vi "custom_operation_461nm_freq.vi"(10 "Channel":T1={"Operation"=0, "Num. Steps"=0, "Begin"=0.0, "Step Size"=0.0, "Input - A"=0, "Input - B"=0, "Output - LO"=0.0, "Output - HI"=0.0, "Reset"=FALSE, "Analog Output"=0, "Trigger Input"=0, "Initialize To"=0, "Digital Inputs"=[0, 0, 0, 0, 0], "Output Values"=[0.0, 0.0, 0.0, 0.0, 0.0], "Num. Inputs"=4} {"Digital Inputs" items=["DIO0", "DIO1", "DIO2", "DIO3", "DIO4", "DIO5", "DIO6", "DIO7", "DIO8", "DIO9", "DIO10", "DIO11", "DIO12", "DIO13", "DIO14", "DIO15", "DIO16", "DIO17", "DIO18", "DIO19", "DIO20", "DIO21", "DIO22", "DIO23", "DIO24", "DIO25", "DIO26", "DIO27", "DIO28", "DIO29", "DIO30", "DIO31"]; "Initialize To" items=["Zero", "Begin Value"]; "Trigger Input" items=["DIO0", "DIO1", "DIO2", "DIO3", "DIO4", "DIO5", "DIO6", "DIO7", "DIO8", "DIO9", "DIO10", "DIO11", "DIO12", "DIO13", "DIO14", "DIO15", "DIO16", "DIO17", "DIO18", "DIO19", "DIO20", "DIO21", "DIO22", "DIO23", "DIO24", "DIO25", "DIO26", "DIO27", "DIO28", "DIO29", "DIO30", "DIO31"]; "Analog Output" items=["AO\\00", "AO\\01", "AO\\02", "AO\\03", "AO\\04", "AO\\05", "AO\\06", "AO\\07", "AO\\08", "AO\\09", "AO\\10", "AO\\11", "AO\\12", "AO\\13", "AO\\14", "AO\\15"]; "Input - B" items=["DIO0", "DIO1", "DIO2", "DIO3", "DIO4", "DIO5", "DIO6", "DIO7", "DIO8", "DIO9", "DIO10", "DIO11", "DIO12", "DIO13", "DIO14", "DIO15", "DIO16", "DIO17", "DIO18", "DIO19", "DIO20", "DIO21", "DIO22", "DIO23", "DIO24", "DIO25", "DIO26", "DIO27", "DIO28", "DIO29", "DIO30", "DIO31"]; "Input - A" items=["DIO0", "DIO1", "DIO2", "DIO3", "DIO4", "DIO5", "DIO6", "DIO7", "DIO8", "DIO9", "DIO10", "DIO11", "DIO12", "DIO13", "DIO14", "DIO15", "DIO16", "DIO17", "DIO18", "DIO19", "DIO20", "DIO21", "DIO22", "DIO23", "DIO24", "DIO25", "DIO26", "DIO27", "DIO28", "DIO29", "DIO30", "DIO31"]; "Operation" items=["OFF", "SWITCH", "AND GATE", "OR GATE", "ITERATION", "CUSTOM - 461nm Freq."]}, 11 "Digital Input Value Array":bool[](array[boolean])=[FALSE, FALSE, FALSE, FALSE, FALSE, FALSE, FALSE, FALSE, FALSE, FALSE, FALSE, FALSE, FALSE, FALSE, FALSE, FALSE, FALSE, FALSE, FALSE, FALSE, FALSE, FALSE, FALSE, FALSE, FALSE, FALSE, FALSE, FALSE, FALSE, FALSE, FALSE, FALSE]) -> (3 "AO Out":fxp<+/-,20,5>)   [LabVIEW 2016]
uses:
  fpga_array_element.ctl
panel:
  # "Boolean Operation Controls"
  # "Iteration Operation Controls"
  # "Custom Operation Controls"
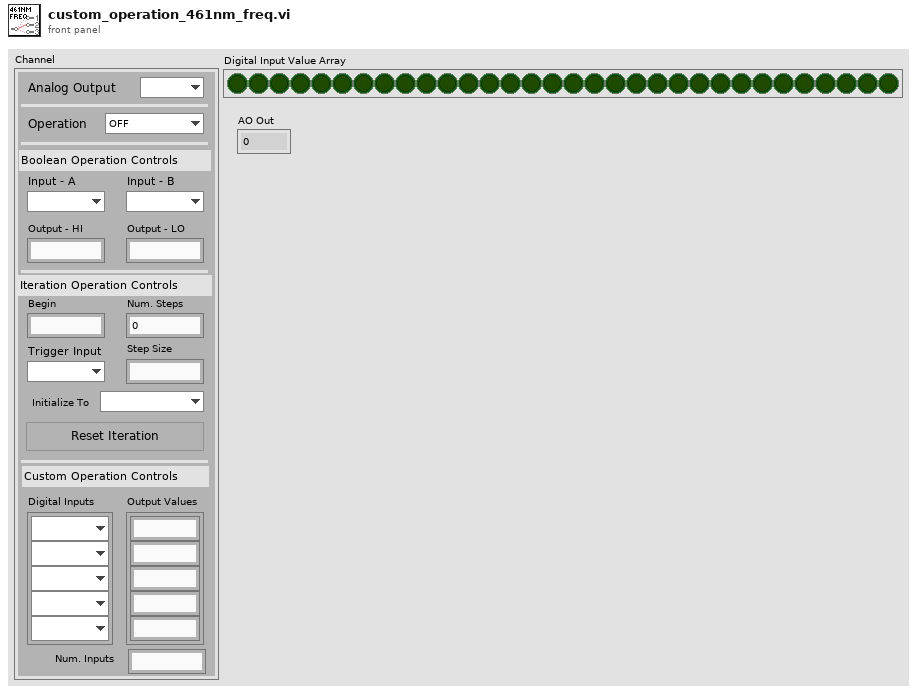
[diagram p1: front panel]
types:
  T1 = typedef "fpga_array_element.ctl" = cluster{"Operation":i16, "Num. Steps":u16, "Begin":fxp<+/-,20,5>, "Step Size":fxp<+/-,20,5>, "Input - A":i32, "Input - B":i32, "Output - LO":fxp<+/-,20,5>, "Output - HI":fxp<+/-,20,5>, "Reset":bool, "Analog Output":i32, "Trigger Input":i32, "Initialize To":i16, "Digital Inputs":i32[], "Output Values":fxp<+/-,20,5>[], "Num. Inputs":u16}
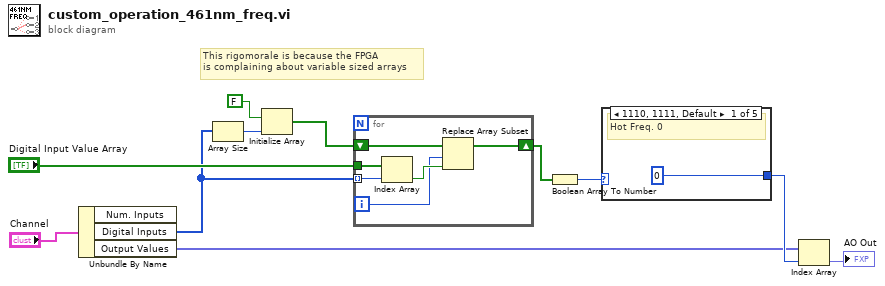
[diagram p0: block diagram]
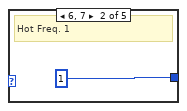
[diagram p2: hidden frame]
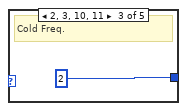
[diagram p3: hidden frame]
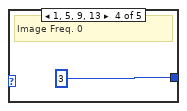
[diagram p4: hidden frame]
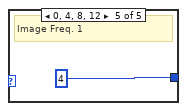
[diagram p5: hidden frame]
diagram:
  # "This rigomorale is because the FPGA\nis complaining about variable sized arrays"
  n1 = Unbundle By Name("Channel") -> ("Digital Inputs"=w5:i32[], "Output Values"=w7:fxp<+/-,20,5>[])  [unwired: 1 out]
  n2 = Array Size(array=w5) -> (size(s)=w4:i32)
  n3 = Initialize Array(FALSE, w4) -> (w2:bool[])
  n4 = for {
    tunnel: "Digital Input Value Array" -> [w17]
    tunnel: w5 -> [w16] mode=indexing
    shift-right: [w12] -> w1
    shift-left: w2 -> [w13]
    i -> [w14]
    n5 = Index Array(array=w17, index=w16) -> (element=w15:bool)
    n6 = Replace Array Subset(array=w13, new element=w15, index=w14) -> (w12:bool[])
  }
  n7 = Boolean Array To Number(Boolean array=w1) -> (number=w9:u32)
  n8 = case shown="1110, 1111, Default" w9 {
    tunnel: [i16 0 i16 1 i16 2 i16 3 i16 4] -> w8
    frame 14, 15, Default {
      # "Hot Freq. 0"
    }
    frame 6, 7 {
      # "Hot Freq. 1"
    }
    frame 2, 3, 10, 11 {
      # "Cold Freq."
    }
    frame 1, 5, 9, 13 {
      # "Image Freq. 0"
    }
    frame 0, 4, 8, 12 {
      # "Image Freq. 1"
    }
  }
  n9 = Index Array(array=w7, index=w8) -> (element=→"AO Out":fxp<+/-,20,5>)
